vi "Configure Carrier Signal.vi"(0 "VISA resource name":refnum<visa-resource-name>, 1 "Carrier Frequency (50 Mhz)":dbl=50000000.0 format="%^#_6g", 2 "Search Span (10 Khz)":dbl=10000.0 format="%^#_6g", 4 "Signal Tracking Method (0: Off)":i32(ring) items=["Off", "Interval", "Tolerance", "Interval & Tolerance"], 5 "error in (no error)":errorcluster, 6 "Automatic Carrier Search (T: Enable)":bool=TRUE, 7 "Drift Span (10 %)":dbl=10.0, 8 "Search Maximum Time (30000)":u32=30000, 9 "Tracking Interval (10 Measurements)":dbl=10.0, 11 "Tolerance (10 dBc/Hz)":dbl=10.0) -> (14 "VISA resource name out":refnum<visa-resource-name>, 19 "error out":errorcluster)   [LabVIEW 2014, in "Agilent ESA PSA Series.lvlib"]
doc: "Configures the carrier signal properties.\n\n<B>Note:</B>\n\nPlease remember that if the <B>Automatic Carrier Search</B> function can not locate the input signal or <B>the Carrier Frequency</B> that you entered is wrong, then the device will send out an error message saying that a carrier wasn't found and continuing the measurement attempts will result in a querry unterminated message.\n\nThis VI is only valid in Phase Noise personality. Use <B>Switch Personality</B> VI to switch to Phase Noise before calling this VI."
uses:
  Agilent ESA PSA Series.lvlib
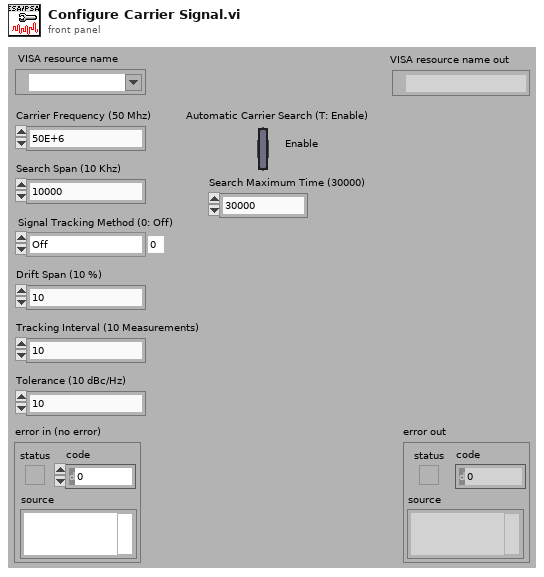
[diagram p1: front panel]
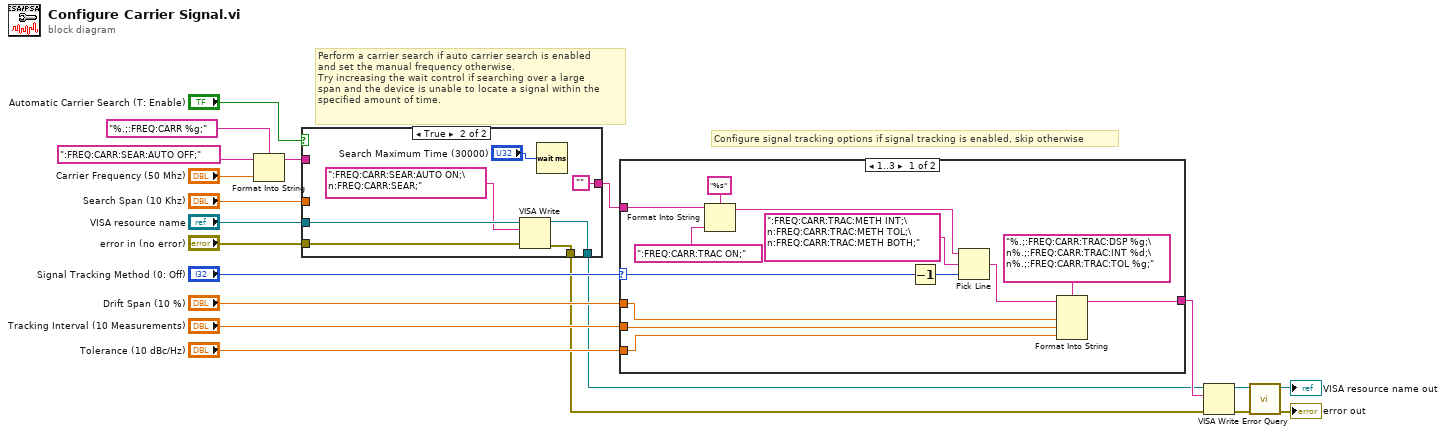
[diagram p0: block diagram]
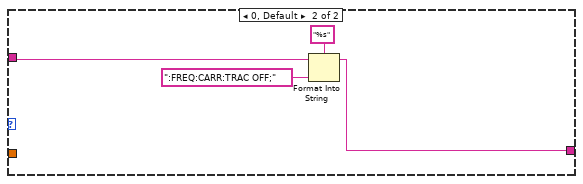
[diagram p2: hidden frame]
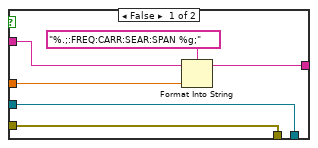
[diagram p3: hidden frame]
diagram:
  # "Configure signal tracking options if signal tracking is enabled, skip otherwise"
  # "Perform a carrier search if auto carrier search is enabled\nand set the manual frequency otherwise.\nTry increasing the wait control if searching over a large\nspan and the device is unable to locate a signal within the \nspecified amount of time."
  n1 = Format Into String(format string="%.;:FREQ:CARR %g;", initial string=":FREQ:CARR:SEAR:AUTO OFF;", "Carrier Frequency (50 Mhz)") -> (resulting string=w13:string)  [unwired: 1 in, 1 out]
  n2 = case shown="True" "Automatic Carrier Search (T: Enable)" {
    tunnel: [w24 ""] -> w11
    tunnel: "Search Span (10 Khz)" -> [w26 _]
    tunnel: w13 -> [w23 _]
    tunnel: "VISA resource name" -> [w22 w33]
    tunnel: "error in (no error)" -> [w21 w32]
    tunnel: [w22 w29] -> w2
    tunnel: [w21 w28] -> w1
    frame False {
      n3 = Format Into String(format string="%.;:FREQ:CARR:SEAR:SPAN %g;", initial string=w23, w26) -> (resulting string=w24:string)  [unwired: 1 in, 1 out]
    }
    frame True {
      n4 = VISA Write(VISA resource name=w33, write buffer=":FREQ:CARR:SEAR:AUTO ON;\n:FREQ:CARR:SEAR;", error in (no error)=w32) -> (VISA resource name out=w29:refnum<visa-resource-name>, error out=w28:errorcluster)  [unwired: 1 out]
      n5 = Wait (ms)(milliseconds to wait="Search Maximum Time (30000)") -> ()  [unwired: 1 out]
    }
  }
  n6 = case shown="1..3" "Signal Tracking Method (0: Off)" {
    selector: "Signal Tracking Method (0: Off)" -> [w38 _]
    tunnel: w11 -> [w43 w50]
    tunnel: [w34 w47] -> w7
    tunnel: "Drift Span (10 %)" -> [w46 _]
    tunnel: "Tracking Interval (10 Measurements)" -> [w36 _]
    tunnel: "Tolerance (10 dBc/Hz)" -> [w35 _]
    frame 1..3 {
      n7 = Format Into String(format string="%s", initial string=w43, ":FREQ:CARR:TRAC ON;" ("input 1")) -> (resulting string=w40:string)  [unwired: 1 in, 1 out]
      n8 = Decrement(x=w38) -> (x-1=w39:i32)
      n9 = Pick Line(string ("")=w40, multi-line string=":FREQ:CARR:TRAC:METH INT;\n:FREQ:CARR:TRAC:METH TOL;\n:FREQ:CARR:TRAC:METH BOTH;", line index=w39) -> (output string=w37:string)
      n10 = Format Into String(format string="%.;:FREQ:CARR:TRAC:DSP %g;\n%.;:FREQ:CARR:TRAC:INT %d;\n%.;:FREQ:CARR:TRAC:TOL %g;", initial string=w37, w46, w36, w35) -> (resulting string=w34:string)  [unwired: 1 in, 1 out]
    }
    frame 0, Default {
      n11 = Format Into String(format string="%s", initial string=w50, ":FREQ:CARR:TRAC OFF;") -> (resulting string=w47:string)  [unwired: 1 in, 1 out]
    }
  }
  n12 = VISA Write(VISA resource name=w2, write buffer=w7, error in (no error)=w1) -> (VISA resource name out=w20:refnum<visa-resource-name>, error out=w19:errorcluster)  [unwired: 1 out]
  n13 = call "Error Query.vi"("error in (no error)"=w19, "VISA resource name"=w20) -> ("error out"=→"error out":errorcluster, "VISA resource name out"=→"VISA resource name out":refnum<visa-resource-name>)  [unwired: 6 in, 2 out]
